vi "Sets_Union(VI-REF).vi"(8 "error in (no error)":errorcluster caption="错误输入（无错误）", 10 "输入数组B":refnum<vi>[](array[refnum]), 11 "输入数组A":refnum<vi>[](array[refnum])) -> (0 "error out":errorcluster caption="错误输出", 3 "输出数组C":refnum<vi>[](array[refnum]))   [LabVIEW 2011]
uses:
  Sets_Unique(VI-REF).vi
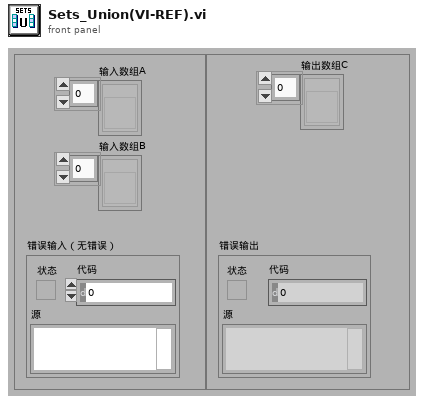
[diagram p1: front panel]
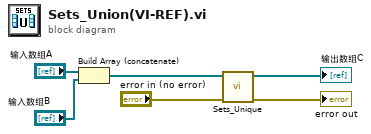
[diagram p0: block diagram]
diagram:
  n1 = Build Array (concatenate)("输入数组A", "输入数组B") -> (w3:refnum<vi>[])
  n2 = call-poly "Sets_Unique.vi"("error in (no error)"="error in (no error)", "输入数组"=w3) -> ("error out"=→"error out":errorcluster, "输出数组"=→"输出数组C":refnum<vi>[])  [unwired: 7 in, 1 out]
